vi "Read Build Number XML Prop Name.vi"(8 "error in (no error)":errorcluster, 11 "NI Build Specification_LV in":refnum<class "NI Build Specification_LV.lvclass">) -> (0 "error out":errorcluster, 2 "Build Number XML Prop Name":string, 3 "NI Build Specification_LV out":refnum<class "NI Build Specification_LV.lvclass">)   [LabVIEW 2017, in "CL_G3_VIComponentBuilder.lvlib" / "NI Build Specification_LV.lvclass"]
uses:
  NI Build Specification_LV.lvclass
  NI Build Specification_LV.lvclass/NI Build Specification_LV.ctl
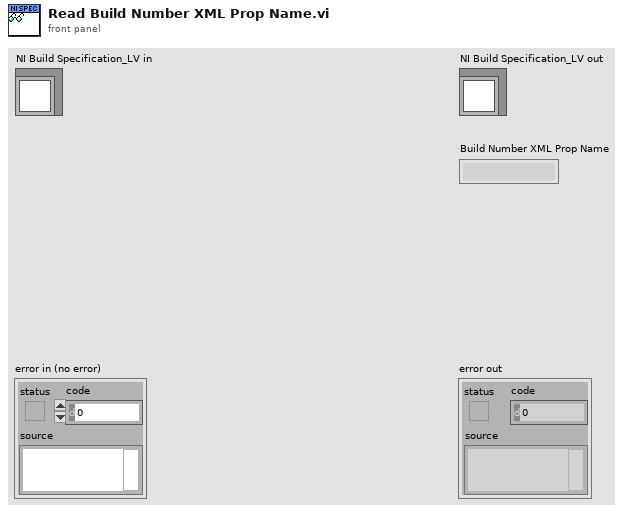
[diagram p1: front panel]
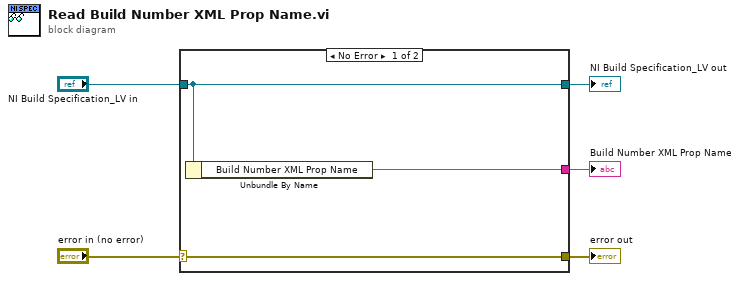
[diagram p0: block diagram]
diagram:
  n1 = case shown="No Error" "error in (no error)" {
    selector: "error in (no error)" -> [w8 w9]
    tunnel: [w8 w9] -> w4
    tunnel: [w7 w10] -> w2
    tunnel: "NI Build Specification_LV in" -> [w7 w10]
    tunnel: [w6 _] -> w1
    frame No Error {
      n2 = Unbundle By Name(w7) -> ("Build Number XML Prop Name"=w6:string)
    }
    frame Error {
    }
  }
  "error out" <- w4
  "NI Build Specification_LV out" <- w2
  "Build Number XML Prop Name" <- w1
